vi "RedOrGreen.vi"(1 "success":bool) -> (0 "color":string)   [LabVIEW 2012]
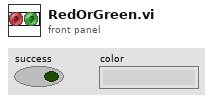
[diagram p1: front panel]
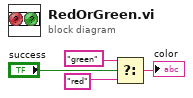
[diagram p0: block diagram]
diagram:
  n1 = Select(t="green" ("format string"), s="success", f="red" ("format string")) -> (s? t:f=→"color":string)
